vi "Andor_Acquire_Im.vi"(4 "AccDoneRef":refnum<vi>, 5 "IntegTime":u32=100 caption="Integration\nTime (ms)" min=1 max=100000 step=1, 6 "Stop Acq":refnum<vi>, 7 "Accumulation":u16=1 min=1 max=256 step=1, 8 "ErrorIn(NoErr)":errorcluster, 9 "Save":bool, 10 "AndorOpQ":refnum<queue>, 11 "AndorAcqQ":refnum<queue>) -> (0 "error out":errorcluster, 1 "Delta(ms)":u32, 2 "DeltaT":u32[](array[numeric]), 3 "Data out":i32[][](array[numeric]))   [LabVIEW 2019]
uses:
  Programmes Labview/LabscanV1A/DevicesClass/InstrumentsClass/AndorSpectro/AndorAcq_States.ctl
  <userlib>/atmcd32d.llb/Error Code Enum typedef.ctl
panel:
  in  "size":i32=262144
  out "AccDone":i32
  out "AcqDone":bool
  in  "Stop Acq":bool
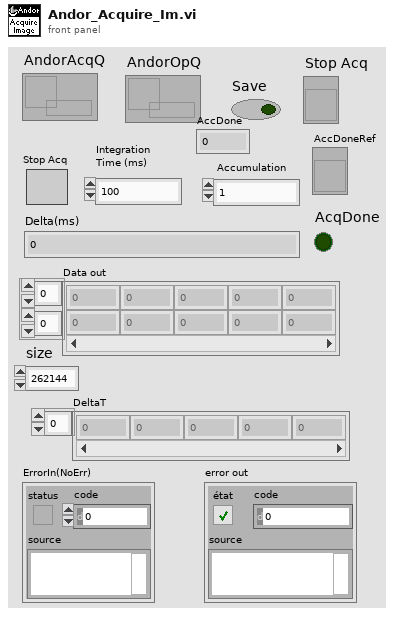
[diagram p1: front panel]
types:
  T1 = typedef "AndorAcq_States.ctl" = enum16{"Start", "Get Status", "GetStatusMulti", "Abort", "Error", "GetData"}
  T2 = typedef "Error Code Enum typedef.ctl" = enum32{"N/A (0)", "DRV_ERROR_CODES", "DRV_SUCCESS", "DRV_VXDNOTINSTALLED", "DRV_ERROR_SCAN", "DRV_ERROR_CHECK_SUM", "DRV_ERROR_FILELOAD", "DRV_UNKNOWN_FUNC", "DRV_ERROR_VXD_INIT", "DRV_ERROR_ADDRESS", "DRV_ERROR_PAGELOCK", "DRV_ERROR_PAGEUNLOCK", "DRV_ERROR_BOARDTEST", "DRV_ERROR_ACK", "DRV_ERROR_UP_FIFO", "DRV_ERROR_PATTERN", "N/A (16)", "DRV_ACQUISITION_ERRORS", "DRV_ACQ_BUFFER", "DRV_ACQ_DOWNFIFO_FULL", "DRV_PROC_UNKONWN_INSTRUCTION", "DRV_ILLEGAL_OP_CODE", "DRV_KINETIC_TIME_NOT_MET", "DRV_ACCUM_TIME_NOT_MET", "DRV_NO_NEW_DATA", "N/A (25)", "DRV_SPOOLERROR", "N/A (27)", "N/A (28)", "N/A (29)", "N/A (30)", "N/A (31)", "N/A (32)", "DRV_TEMPERATURE_CODES", "DRV_TEMPERATURE_OFF", "DRV_TEMPERATURE_NOT_STABILIZED", "DRV_TEMPERATURE_STABILIZED", "DRV_TEMPERATURE_NOT_REACHED", "DRV_TEMPERATURE_OUT_RANGE", "DRV_TEMPERATURE_NOT_SUPPORTED", "DRV_TEMPERATURE_DRIFT", "N/A (41)", "N/A (42)", "N/A (43)", "N/A (44)", "N/A (45)", "N/A (46)", "N/A (47)", "N/A (48)", "DRV_GENERAL_ERRORS", "DRV_INVALID_AUX", "DRV_COF_NOTLOADED", "DRV_FPGAPROG", "DRV_FLEXERROR", "DRV_GPIBERROR", "N/A (55)", "N/A (56)", "N/A (57)", "N/A (58)", "N/A (59)", "N/A (60)", "N/A (61)", "N/A (62)", "N/A (63)", "DRV_DATATYPE", "DRV_DRIVER_ERRORS", "DRV_P1INVALID", "DRV_P2INVALID", "DRV_P3INVALID", "DRV_P4INVALID", "DRV_INIERROR", "DRV_COFERROR", "DRV_ACQUIRING", "DRV_IDLE", "DRV_TEMPCYCLE", "DRV_NOT_INITIALIZED", "DRV_P5INVALID", "DRV_P6INVALID", "DRV_INVALID_MODE", "DRV_INVALID_FILTER", "DRV_I2CERRORS", "DRV_I2CDEVNOTFOUND", "DRV_I2CTIMEOUT", "DRV_P7INVALID", "N/A (84)", "N/A (85)", "N/A (86)", "N/A (87)", "N/A (88)", "N/A (89)", "DRV_IOCERROR", "DRV_VRMVERSIONERROR"}
  T3 = cluster{"Message":string, "Data":variant, "Code":i32}
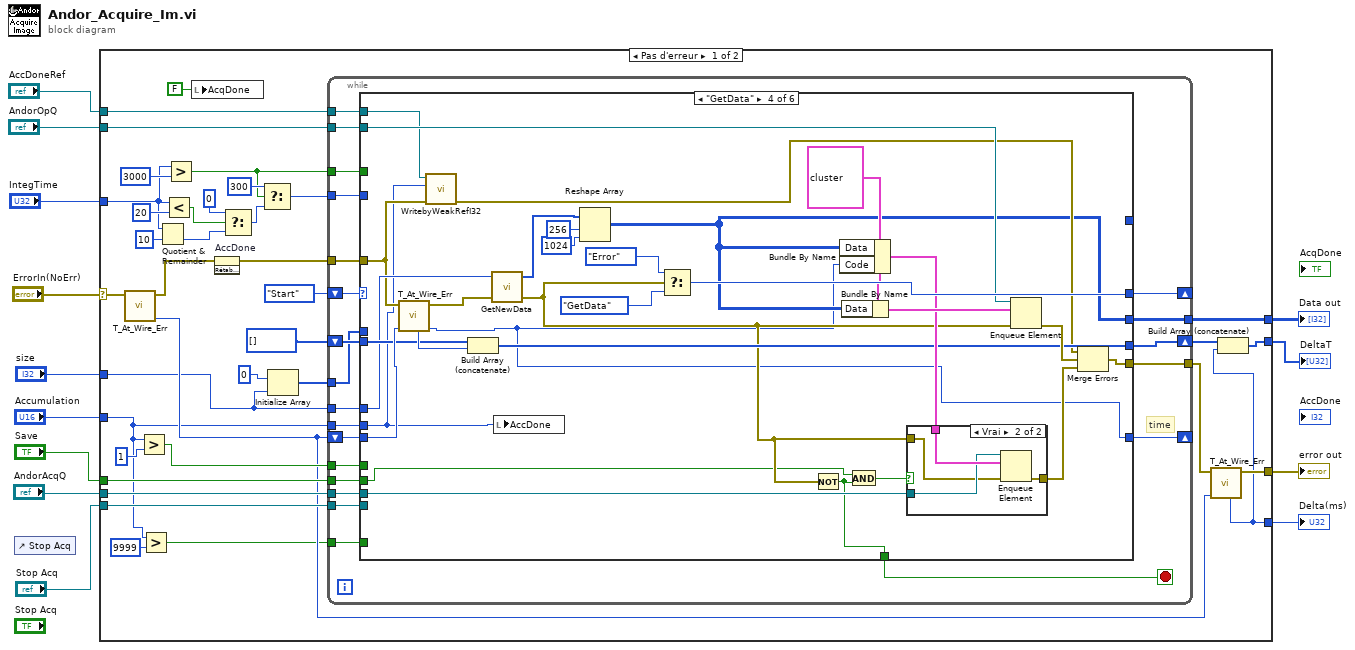
[diagram p0: block diagram]
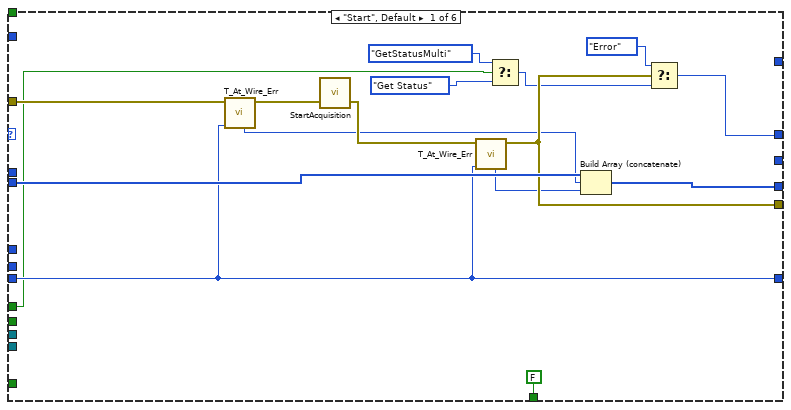
[diagram p2: hidden frame]
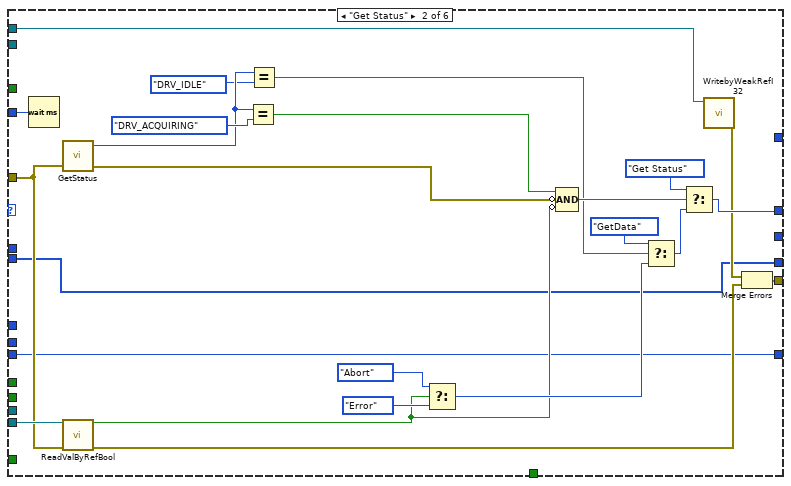
[diagram p3: hidden frame]
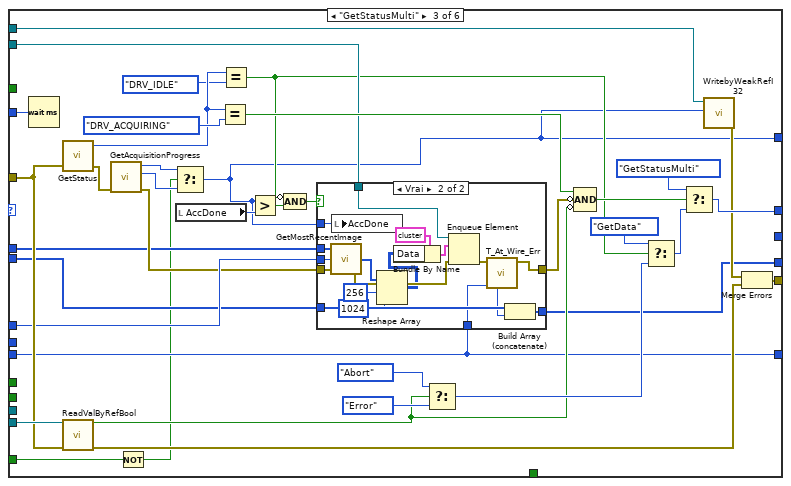
[diagram p4: hidden frame]
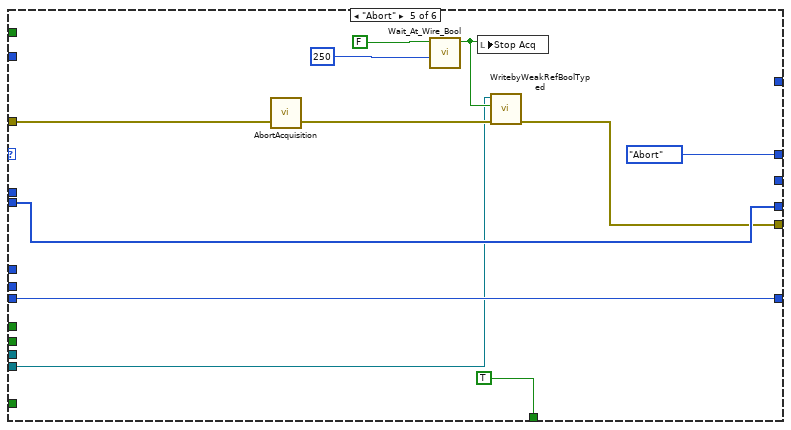
[diagram p7: hidden frame]
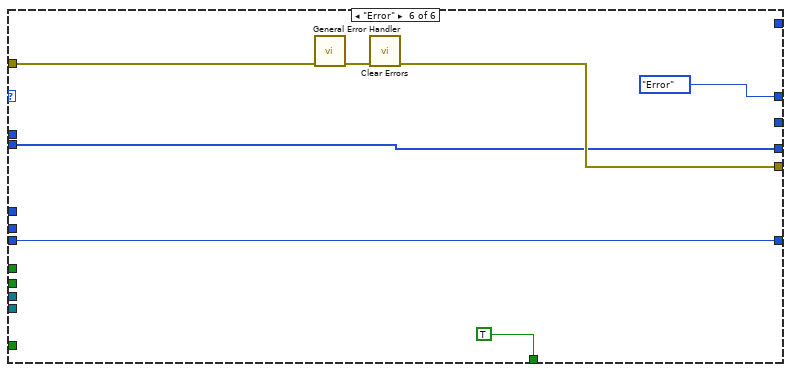
[diagram p8: hidden frame]
diagram:
  n1 = control-ref of="Stop Acq"() -> ()  [unwired: 1 out]
  n2 = case shown="Pas d'erreur" "ErrorIn(NoErr)" {
    selector: "ErrorIn(NoErr)" -> [w38 w224]
    tunnel: [w36 w224] -> w12
    tunnel: "AndorAcqQ" -> [w49 _]
    tunnel: "AndorOpQ" -> [w48 _]
    tunnel: "Save" -> [w47 _]
    tunnel: "Accumulation" -> [w16 _]
    tunnel: "Stop Acq" -> [w46 _]
    tunnel: "IntegTime" -> [w29 _]
    tunnel: [w24 _] -> w5
    tunnel: [w18 _] -> w4
    tunnel: [w17 _] -> w3
    tunnel: "AccDoneRef" -> [w34 _]
    tunnel: "size" -> [w23 _]
    frame No Error {
      n3 = call <userlib>:"T_At_Wire_Err.vi"("error in (no error)"=w38) -> ("Clock(ms)"=w35:u32, "error out"=w32:errorcluster)  [unwired: 8 in, 1 out]
      n4 = Greater?(x=w16, y=u16 1) -> (0:w42:bool)
      n5 = Greater?(x=w16, y=u16 9999) -> (0:w14:bool)
      n6 = Quotient & Remainder(x=w29, y=u32 10) -> (floor(x/y)=w25:u32)  [unwired: 1 out]
      n7 = Less?(x=w29, y=u32 20 ("limite supérieure")) -> (x < y?=w40:bool)
      n8 = Greater?(x=w29, y=u32 3000 ("limite supérieure")) -> (0:w20:bool)
      n9 = local write "AcqDone"(FALSE ("AcqDone")) -> ()
      n10 = invoke on="AccDone" class="NumNb (strict)" method="RétablirValParDéfaut"(error in=w32) -> (error out=w31:errorcluster)  [unwired: 2 in, 2 out]
      n11 = Select(t=u32 0 ("cas vrai"), s=w40, f=w25) -> (s? t:f=w28:u32)
      n12 = Select(t=u32 300 ("cas vrai"), s=w20, f=w28) -> (s? t:f=w26:u32)
      n13 = Initialize Array(0, w23) -> (w21:i32[])
      n14 = while {
        tunnel: [w72] -> w37
        tunnel: w31 -> [w70]
        shift-right: [w69] -> _
        shift-left: AndorAcq_States."Start" ("AndorAcqSt") -> [w71]
        tunnel: w48 -> [w67]
        tunnel: w49 -> [w66]
        tunnel: w47 -> [w65]
        tunnel: w16 -> [w64]
        tunnel: w46 -> [w63]
        tunnel: w26 -> [w62]
        tunnel: w42 -> [w61]
        shift-right: [w57] -> _
        shift-left: w35 -> [w60]
        shift-right: [w59] -> w19
        shift-left: u32[] [] -> [w58]
        tunnel: w34 -> [w56]
        tunnel: w23 -> [w55]
        tunnel: [w54] -> w24
        tunnel: w21 -> [w53]
        tunnel: w20 -> [w52]
        tunnel: w14 -> [w51]
        stop <- w68 stop-if-true
        # "time"
        n15 = case shown="\"GetData\"" w71 {
          tunnel: [w83 w97 w135 w196 w206 w219] -> w72
          tunnel: w70 -> [w80 w98 w136 w182 w216 w223]
          tunnel: [w87 w110 w148 w200 AndorAcq_States."Abort" ("AndorAcqSt") AndorAcq_States."Error" ("AndorAcqSt")] -> w69
          tunnel: [FALSE _ _ w171 TRUE TRUE] -> w68
          tunnel: w67 -> [_ _ w127 w189 _ _]
          tunnel: w66 -> [_ _ _ w198 _ _]
          tunnel: w65 -> [_ _ _ w172 _ _]
          tunnel: w64 -> [_ _ _ w181 _ _]
          tunnel: w63 -> [_ w99 w137 _ w207 _]
          tunnel: w62 -> [_ w100 w138 _ _ _]
          tunnel: w61 -> [w76 _ _ _ _ _]
          tunnel: [w77 w91 w118 w174 w209 w218] -> w57
          tunnel: w60 -> [w77 w91 w118 w190 w209 w218]
          tunnel: [w82 w89 w119 w187 w208 w217] -> w59
          tunnel: w58 -> [w85 w89 w120 w186 w208 w217]
          tunnel: w56 -> [_ w96 w134 w180 _ _]
          tunnel: [_ _ w114 _ _ _] -> _
          tunnel: w55 -> [_ _ w130 w185 _ _]
          tunnel: [_ _ _ w177 _ _] -> w54
          tunnel: w53 -> [_ _ w123 _ _ _]
          tunnel: w52 -> [_ _ _ _ _ _]
          tunnel: w51 -> [_ _ w115 _ _ _]
          frame "Start", Default {
            n16 = call <userlib>:"T_At_Wire_Err.vi"("InitClock(ms)"=w77, "error in (no error)"=w80) -> ("error out"=w79:errorcluster, "Delta(ms)"=w78:u32)  [unwired: 7 in, 1 out]
            n17 = call <userlib>:"StartAcquisition.vi"("error in (no error)"=w79) -> ("error out"=w84:errorcluster)  [unwired: 1 in, 1 out]
            n18 = call <userlib>:"T_At_Wire_Err.vi"("InitClock(ms)"=w77, "error in (no error)"=w84) -> ("error out"=w83:errorcluster, "Delta(ms)"=w81:u32)  [unwired: 7 in, 1 out]
            n19 = Select(t=AndorAcq_States."GetStatusMulti" ("AndorAcqSt"), s=w76, f=AndorAcq_States."Get Status" ("AndorAcqSt")) -> (s? t:f=w73:T1)
            n20 = Build Array (concatenate)(w85, w78, w81) -> (w82:u32[])
            n21 = Select(t=AndorAcq_States."Error" ("AndorAcqSt"), s=w83, f=w73) -> (s? t:f=w87:T1)
          }
          frame "Get Status" {
            n22 = Wait (ms)(milliseconds to wait=w100) -> ()  [unwired: 1 out]
            n23 = call <userlib>:"GetStatus.vi"("error in (no error)"=w98) -> ("error out"=w90:errorcluster, "status"=w108:T2)  [unwired: 2 in, 1 out]
            n24 = call <userlib>:"ReadValByRefBool.vi"("Control Ref"=w99, "error in"=w98) -> ("Valeur"=w92:bool, "error out"=w94:errorcluster)  [unwired: 12 in]
            n25 = Equal?(x=w108, y=Error_Code_Enum_typedef."DRV_ACQUIRING" ("status")) -> (x = y?=w111:bool)
            n26 = Equal?(x=w108, y=Error_Code_Enum_typedef."DRV_IDLE" ("status")) -> (x = y?=w93:bool)
            n27 = Select(t=AndorAcq_States."Abort" ("AndorAcqSt"), s=w92, f=AndorAcq_States."Error" ("AndorAcqSt")) -> (s? t:f=w106:T1)
            n28 = Compound Arithmetic op=AND ("Opérateur arithmétique")(w111, invert w90, invert w92) -> (w109:bool)
            n29 = Select(t=AndorAcq_States."GetData" ("AndorAcqSt"), s=w93, f=w106) -> (s? t:f=w105:T1)
            n30 = Select(t=AndorAcq_States."Get Status" ("AndorAcqSt"), s=w109, f=w105) -> (s? t:f=w110:T1)
            n31 = call <userlib>:"WritebyWeakRefI32.vi"("Control Ref"=w96) -> ("error out"=w95:errorcluster)  [unwired: 10 in]
            n32 = Merge Errors(w95, w94) -> (w97:errorcluster)
          }
          frame "GetStatusMulti" {
            n33 = Wait (ms)(milliseconds to wait=w138) -> ()  [unwired: 1 out]
            n34 = call <userlib>:"GetStatus.vi"("error in (no error)"=w136) -> ("error out"=w129:errorcluster, "status"=w146:T2)  [unwired: 2 in, 1 out]
            n35 = call <userlib>:"ReadValByRefBool.vi"("Control Ref"=w137, "error in"=w136) -> ("Valeur"=w122:bool, "error out"=w132:errorcluster)  [unwired: 12 in]
            n36 = call <userlib>:"GetAcquisitionProgress.vi"("error in (no error)"=w129) -> ("error out"=w128:errorcluster, "series"=w116:i32, "accum"=w117:i32)  [unwired: 3 in, 1 out]
            n37 = Not(x=w115) -> (.not. x?=w113:bool)
            n38 = Select(t=w117, s=w113, f=w116) -> (s? t:f=w114:i32)
            n39 = local read "AccDone"() -> (w131:i32)
            n40 = Equal?(x=w146, y=Error_Code_Enum_typedef."DRV_ACQUIRING" ("status")) -> (x = y?=w149:bool)
            n41 = Equal?(x=w146, y=Error_Code_Enum_typedef."DRV_IDLE" ("status")) -> (x = y?=w124:bool)
            n42 = Greater?(x=w114, y=w131) -> (0:w126:bool)
            n43 = Compound Arithmetic op=AND ("Opérateur arithmétique")(invert w124, w126) -> (w125:bool)
            n44 = case shown="Vrai" w125 {
              tunnel: w130 -> [_ w170]
              tunnel: w128 -> [w152 w169]
              tunnel: w127 -> [_ w166]
              tunnel: [w152 w161] -> w121
              tunnel: w123 -> [_ w165]
              tunnel: w114 -> [_ w164]
              tunnel: w120 -> [w151 w160]
              tunnel: [w151 w158] -> w119
              tunnel: w118 -> [_ w157]
              frame False {
              }
              frame True {
                n45 = call <userlib>:"GetMostRecentImage.vi"("error in (no error)"=w169, "size"=w170, "array"=w165) -> ("error out"=w163:errorcluster, "array"=w156:i32[])  [unwired: 1 out]
                n46 = local write "AccDone"(w164) -> ()
                n47 = Reshape Array(w156, 256 ("taille de la dimension"), 1024 ("taille de la dimension")) -> (w153:i32[][])
                n48 = Bundle By Name(cluster=T3 {"Message"="PlotImg", "Data"=variant, "Code"=1}, "Data"=w153) -> (w168:T3)
                n49 = Enqueue Element(queue=w166, element=w168, error in (no error)=w163) -> (error out=w162:errorcluster)  [unwired: 1 in, 2 out]
                n50 = call <userlib>:"T_At_Wire_Err.vi"("InitClock(ms)"=w157, "error in (no error)"=w162) -> ("error out"=w161:errorcluster, "Delta(ms)"=w159:u32)  [unwired: 7 in, 1 out]
                n51 = Build Array (concatenate)(w160, w159) -> (w158:u32[])
              }
            }
            n52 = Select(t=AndorAcq_States."Abort" ("AndorAcqSt"), s=w122, f=AndorAcq_States."Error" ("AndorAcqSt")) -> (s? t:f=w144:T1)
            n53 = Compound Arithmetic op=AND ("Opérateur arithmétique")(w149, invert w121, invert w122) -> (w147:bool)
            n54 = Select(t=AndorAcq_States."GetData" ("AndorAcqSt"), s=w124, f=w144) -> (s? t:f=w143:T1)
            n55 = Select(t=AndorAcq_States."GetStatusMulti" ("AndorAcqSt"), s=w147, f=w143) -> (s? t:f=w148:T1)
            n56 = call <userlib>:"WritebyWeakRefI32.vi"("Valeur"=w114, "Control Ref"=w134) -> ("error out"=w133:errorcluster)  [unwired: 9 in]
            n57 = Merge Errors(w133, w132) -> (w135:errorcluster)
          }
          frame "GetData" {
            w193 = T3 {"Message"="PlotImg", "Data"=variant, "Code"=1}
            n58 = call <userlib>:"T_At_Wire_Err.vi"("InitClock(ms)"=w190, "error in (no error)"=w182) -> ("Clock(ms)"=w174:u32, "error out"=w191:errorcluster, "Delta(ms)"=w188:u32)  [unwired: 7 in]
            n59 = call <userlib>:"WritebyWeakRefI32.vi"("error in"=w182, "Valeur"=w181, "Control Ref"=w180) -> ("error out"=w179:errorcluster)  [unwired: 8 in]
            n60 = Build Array (concatenate)(w186, w188) -> (w187:u32[])
            n61 = call <userlib>:"GetNewData.vi"("error in (no error)"=w191, "size"=w185) -> ("error out"=w183:errorcluster, "array"=w178:i32[])  [unwired: 1 in, 1 out]
            n62 = local write "AccDone"(w181) -> ()
            n63 = Reshape Array(w178, 256 ("taille de la dimension"), 1024 ("taille de la dimension")) -> (w177:i32[][])
            n64 = Select(t=AndorAcq_States."Error" ("AndorAcqSt"), s=w183, f=AndorAcq_States."GetData" ("AndorAcqSt")) -> (s? t:f=w200:T1)
            n65 = Not(x=w183) -> (.not. x?=w171:bool)
            n66 = Bundle By Name(cluster=w193, "Data"=w177, "Code"=w174) -> (w192:T3)
            n67 = Bundle By Name(cluster=w193, "Data"=w177) -> (w197:T3)
            n68 = And(x=w172, y=w171) -> (x .and. y?=w173:bool)
            n69 = case shown="Vrai" w173 {
              tunnel: w198 -> [_ w203]
              tunnel: w192 -> [_ w205]
              tunnel: w183 -> [w201 w202]
              tunnel: [w201 w204] -> w195
              frame False {
              }
              frame True {
                n70 = Enqueue Element(queue=w203, element=w205, error in (no error)=w202) -> (error out=w204:errorcluster)  [unwired: 1 in, 2 out]
              }
            }
            n71 = Enqueue Element(queue=w189, element=w197, error in (no error)=w183) -> (error out=w199:errorcluster)  [unwired: 1 in, 2 out]
            n72 = Merge Errors(w179, w199, w195) -> (w196:errorcluster)
          }
          frame "Abort" {
            n73 = call <userlib>:"AbortAcquisition.vi"("error in (no error)"=w216) -> ("error out"=w211:errorcluster)  [unwired: 1 in, 1 out]
            n74 = call <userlib>:"Wait_At_Wire_Bool.vi"("Wait (ms)"=u32 250, "error in (no error)"=FALSE) -> ("error out"=w210:bool)  [unwired: 7 in, 2 out]
            n75 = local write "Stop Acq"(w210) -> ()
            n76 = call <userlib>:"WritebyWeakRefBoolTyped.vi"("error in"=w211, "Valeur"=w210, "Control Ref"=w207) -> ("error out"=w206:errorcluster)  [unwired: 8 in]
          }
          frame "Error" {
            n77 = call <vilib>:"General Error Handler.vi"("error in (no error)"=w223) -> ("error out"=w222:errorcluster)  [unwired: 10 in, 4 out]
            n78 = call <vilib>:"Clear Errors.vi"("error in (no error)"=w222) -> ("error out"=w219:errorcluster)  [unwired: 5 in, 1 out]
          }
        }
      }
      n79 = call <userlib>:"T_At_Wire_Err.vi"("InitClock(ms)"=w35, "error in (no error)"=w37) -> ("error out"=w36:errorcluster, "Delta(ms)"=w17:u32)  [unwired: 7 in, 1 out]
      n80 = Build Array (concatenate)(w19, w17) -> (w18:u32[])
    }
    frame Error {
    }
  }
  "error out" <- w12
  "Data out" <- w5
  "DeltaT" <- w4
  "Delta(ms)" <- w3
